vi "SWERVE_CALC_CONT_ERROR.vi"(9 "ErrorRange":dbl, 11 "Error":dbl) -> (3 "Continuous Error":dbl)   [LabVIEW 2019]
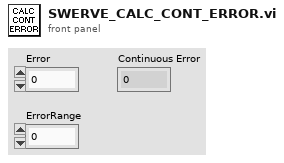
[diagram p1: front panel]
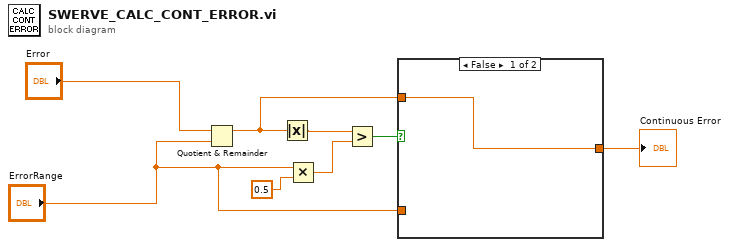
[diagram p0: block diagram]
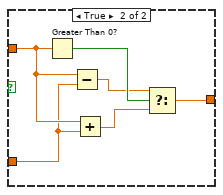
[diagram p2: hidden frame]
diagram:
  n1 = Quotient & Remainder(x="Error", y="ErrorRange") -> (x-y*floor(x/y)=w6:dbl)  [unwired: 1 out]
  n2 = Absolute Value(x=w6) -> (abs(x)=w3:dbl)
  n3 = Multiply(x="ErrorRange", y=0.5) -> (x*y=w4:dbl)
  n4 = Greater?(x=w3, y=w4) -> (0:w5:bool)
  n5 = case shown="False" w5 {
    tunnel: [w9 w10] -> w7
    tunnel: w6 -> [w9 w14]
    tunnel: "ErrorRange" -> [_ w13]
    frame False {
    }
    frame True {
      n6 = Greater Than 0?(x=w14) -> (x > 0?=w15:bool)
      n7 = Subtract(x=w14, y=w13) -> (x-y=w12:dbl)
      n8 = Add(x=w14, y=w13) -> (x+y=w11:dbl)
      n9 = Select(t=w12, s=w15, f=w11) -> (s? t:f=w10:dbl)
    }
  }
  "Continuous Error" <- w7
